vi "Curtin1_Acquire.vi"(8 "MainVI":refnum<vi>, 11 "Settings":T3={"Name of test"="ScratchPad", "Date"=timestamp(0 s since 1904-01-01), "Location"="Home", "Template"="ScratchPad", "Soundcard"="OCTA-CAPTURE", "resolution"=32, "Sampling rate"=48000, "Ch1 Gain "=25.0, "Ch2 Gain"=10.0, "Sample time (s)"=0.3, "Pre-trigger (s)"=0.001, "Hammer Threshold"=10.0, "Positions"=12, "Taps/Position"=5, "Set Names"="H,V", "Freq resolution"=1.0, "Hammer cutoff"=0.025, "Mic cutoff"=0.25, "Double bounce "=10.0, "Hammer Cal"=10.0, "dB Offset"=0.0, "Accel Cal"=10.0, "Vibrometer Cal"=0.0, "Mic Cal"=0.0, "Output"=2, "Voltage Cal"=0.01, "Vibrometer Port"="ASRL27::INSTR", "Range"=4, "High Pass"=2, "Bandwidth"=4, "X Range"=[], "Y Range"=[], "dB Spread"=0.0, "Trigger"=0, "Ch_1"=25, "Ch_2"=25, "flip?"=FALSE, "60Hz"=FALSE, "Time offset"=0.0, "Piezo Cal"=1.0, "Default Notes"=""} {"Ch_2" min=1 step=1; "Ch_1" min=1 max=100 step=1; "Trigger" items=["Hammer (force)", "Self-tap", "Spacebar"]; "Bandwidth" items=["1 kHz"=1, "5 kHz"=5, "10 kHz"=10, "25 kHz"=25, "50 kHz"=50, "100 kHz"=100]; "High Pass" items=["Off", "13 Hz", "104 Hz"]; "Range" items=["10 mm/s"=1, "20 mm/s"=2, "50 mm/s"=5, "100 mm/s"=10, "200 mm/s"=20, "500 mm/s"=50, "1 m/s"=100, "2 m/s"=200]; "Output" items=["Accelerometer", "Speed (from acceleration)", "Microphone", "Vibrometer", "Piezo"]; "Voltage Cal" format="%#_13g"; "Ch2 Gain" format="%#_13g"; "Ch1 Gain" format="%#_13g"; "Double bounce" min=0.0; "Mic cutoff" min=0.0 format="%#_4g"; "Hammer cutoff" min=0.0 format="%#_4g"; "Freq resolution" min=0.0; "Pre-trigger (s)" format="%#_13g"; "Date" format="%<%H:%M\n%d/%m/%y>T"; "resolution" items=["16 bit"=16, "24 bit"=24, "32 bit"=32]; "Sampling rate" items=["22050 samp/s"=22050, "44100 samp/s"=44100, "48000 samp/s"=48000]}) -> (1 "Name Change?":bool, 2 "Data?":bool, 3 "Average FRF":cluster{dbl, "df":dbl, dbl[]}[](graph))   [LabVIEW 2022 SP3]
uses:
  AmpCtrl.ctl
  PreferencesControl.ctl
  <extravilib>/ChannelInstances/Lossy Stream-a[.](wfm(dbl))/EndpointRead.vi
  Mic/Mic_Global.vi
  <extravilib>/ChannelInstances/Lossy Stream-a[.](wfm(dbl))/Instantiate.vi
  <extravilib>/ChannelInstances/Tag-a[.](wfm(dbl))/Instantiate.vi
  <extravilib>/ChannelInstances/Tag-a[.](wfm(dbl))/EndpointRead.vi
  <extravilib>/ChannelInstances/Lossy Stream-a[.](wfm(dbl))/)Channel.vi
  <resource>/ChannelSupport/_ChannelSupport/WaitIfNeeded.vi
  <extravilib>/ChannelInstances/Tag-a[.](wfm(dbl)).lvlib
  <extravilib>/ChannelInstances/Lossy Stream-a[.](wfm(dbl)).lvlib
panel:
  in  "Record Button":bool=TRUE
  in  "Tab Control":enum32{"graphs", "settings", "Notes"}(tab)
  in  "Move":bool
  in  "Motor Settings":bool
  in  "Tap":bool
  in  "Method":enum16{"Sqrt(H1H2)", "H1", "H2"}(ring)
  in  "History":bool=TRUE
  in  "Help":bool
  in  "Beam":bool
  in  "rescale Y Axes":bool
  in  "Open Sound":bool
  in  "View":u16(ring) items=["Raw", "Volts", "Units (Pa, N, etc)"]
  out "Hammer Spectrum":cluster{dbl, "df":dbl, "FFT {X}":dbl[]}[](graph)
  out "Hammer Data":cluster{dbl, "dt":dbl, "Y":dbl[]}[](graph)
  out "Microphone Data":cluster{dbl, "dt":dbl, "Y":dbl[]}[](graph)
  out "Volume":T1 {"Mic" scale=0.0..100.0; "Hammer" scale=0.0..100.0}
  in  "OpenVibrometer":bool
  in  "New":bool
  in  "Save SP":bool
  in  "Export":bool
  in  "Plot View":T2={"Alerts"=FALSE, "Log X Axis"=TRUE, "dB scale"=TRUE, "Averaging"=TRUE, "Fade"=0.0, "Centroids?"=FALSE}
  in  "Locked":bool
  in  "Notes":string
  in  "Done":bool
  out "Progress Bar":picture
  in  "zoom":bool
  in  "dB Spread":dbl=40.0
  in  "rescale Y":bool
  in  "stop":bool
  out "Alarms":string
  # "Hz"
  # "dB"
  # "dB"
  # "sec"
  # "sec"
  # "mV/Pa"
  # "mV/m/s2"
  # "mV/mm/s"
  # "V/N"
  # "sec"
  # "sec"
  # "mV/N"
  # "a.u."
  # "a.u."
  # "sec"
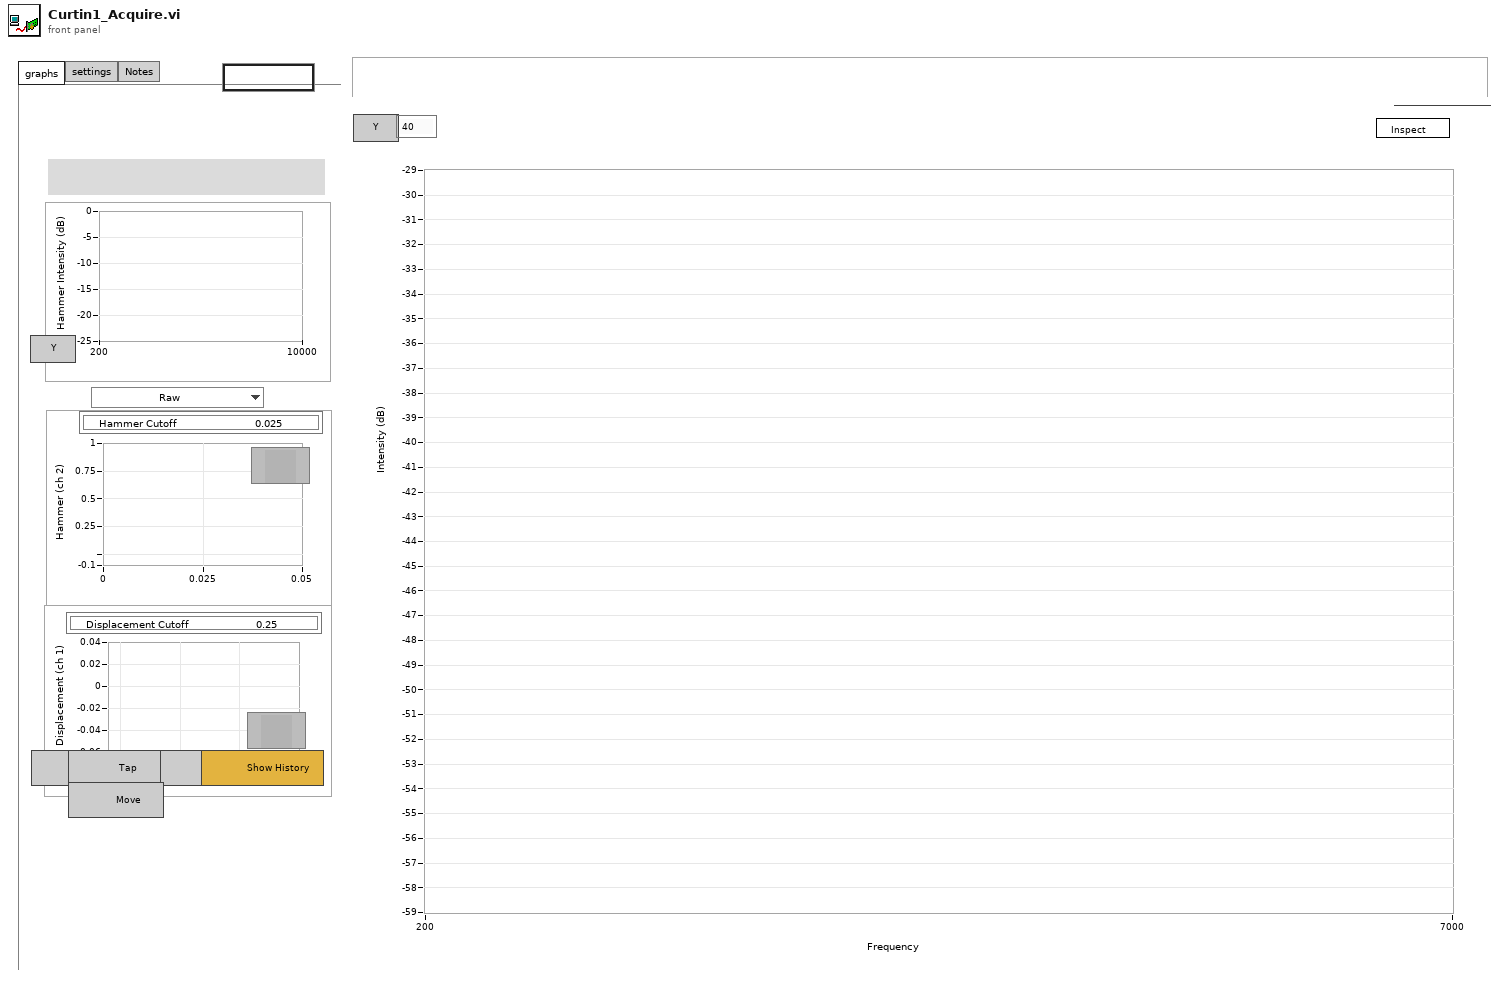
[diagram p1: front panel]
types:
  T1 = typedef "AmpCtrl.ctl" = cluster{"Hammer":u8, "Mic":u8, "Mic In":string}
  T2 = cluster{"Alerts":bool, "Log X Axis":bool, "dB scale":bool, "Averaging":bool, "Fade":dbl, "Centroids?":bool}
  T3 = typedef "PreferencesControl.ctl" = cluster{"Name of test":string, "Date":timestamp, "Location":string, "Template":string, "Soundcard":string, "resolution":u16, "Sampling rate":u16, "Ch1 Gain ":dbl, "Ch2 Gain":dbl, "Sample time (s)":dbl, "Pre-trigger (s)":dbl, "Hammer Threshold":dbl, "Positions":i16, "Taps/Position":i16, "Set Names":string, "Freq resolution":dbl, "Hammer cutoff":dbl, "Mic cutoff":dbl, "Double bounce ":dbl, "Hammer Cal":dbl, "dB Offset":dbl, "Accel Cal":dbl, "Vibrometer Cal":dbl, "Mic Cal":dbl, "Output":u16, "Voltage Cal":dbl, "Vibrometer Port":refnum<visa-resource-name>, "Range":u16, "High Pass":u16, "Bandwidth":u16, "X Range":cluster{"Minimum":dbl, "Maximum":dbl, "Increment":dbl, "Minor Increment":dbl, "Start":dbl}[], "Y Range":cluster{"Minimum":dbl, "Maximum":dbl, "Increment":dbl, "Minor Increment":dbl, "Start":dbl}[], "dB Spread":dbl, "Trigger":u16, "Ch_1":u8, "Ch_2":u8, "flip?":bool, "60Hz":bool, "Time offset":dbl, "Piezo Cal":dbl, "Default Notes":string}
  T4 = enum32{"Invalid", "Standard", "Closed", "Hidden", "Minimized", "Maximized"}
  T5 = enum16{"Initialize", "Free run", "One Shot - waiting", "One Shot - triggered", "Wait", "Close"}
  T6 = enum16{"Always On", "Always Off", "Off While Running"}
  T7 = enum8{"Enabled", "Disabled", "Disabled and Grayed Out"}
  T8 = typedef "Tag-a[.](wfm(dbl)).lvlib/))Channel.ctl" = refnum<queue>
  T9 = typedef "Lossy Stream-a[.](wfm(dbl)).lvlib/)Channel.ctl" = refnum<queue>
  T10 = typedef "LVBoundsTypeDef.ctl" = cluster{"Width":u32, "Height":u32}
  T11 = cluster{"Minimum":dbl, "Maximum":dbl, "Increment":dbl, "Minor Increment":dbl, "Start":dbl}
  T12 = typedef "eventvkey.ctl" = enum16{"ASCII", "Enter", "Return", "Shift", "Ctrl", "Alt", "Cmd", "Opt", "Caps", "NumLock", "Clear", "Break", "Up", "Down", "Left", "Right", "Insert", "Delete", "Home", "End", "PageUp", "PageDown", "Escape", "Help", "Pause", "ScrollLock", "F1", "F2", "F3", "F4", "F5", "F6", "F7", "F8", "F9", "F10", "F11", "F12", "F13", "F14", "F15", "F16", "F17", "F18", "F19", "F20", "F21", "F22", "F23", "F24", "Play", "VolumeUp", "VolumeDown", "Mute", "Two Byte Char"}
  T13 = typedef "LVMouseTypeDef.ctl" = cluster{"Mouse Position":cluster{"X":i32, "Y":i32}, "Mouse Modifiers":cluster{"Button Down":bool, "Shift Mod":bool, "Menu Mod":bool, "Option Mod":bool}}
  T14 = typedef "LVRangeTypeDef.ctl" = cluster{"Minimum":dbl, "Maximum":dbl, "Increment":dbl, "Minor Increment":dbl, "Start":dbl}
  T15 = cluster{"Minimum":dbl, "Maximum":dbl, "Increment":dbl, "Minor Increment":dbl, "Start":dbl}[]
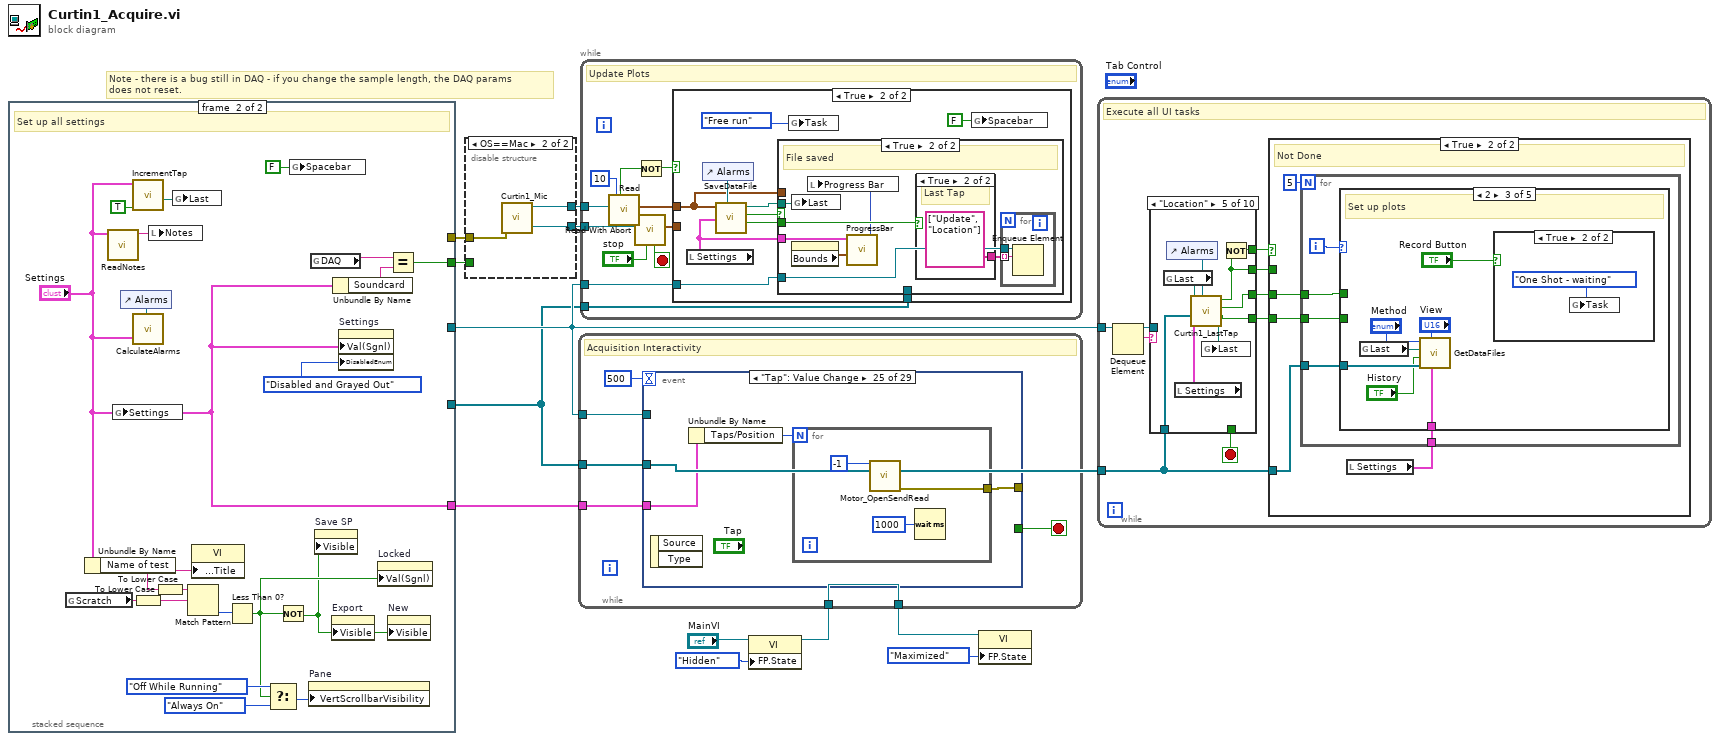
[diagram p0: block diagram]
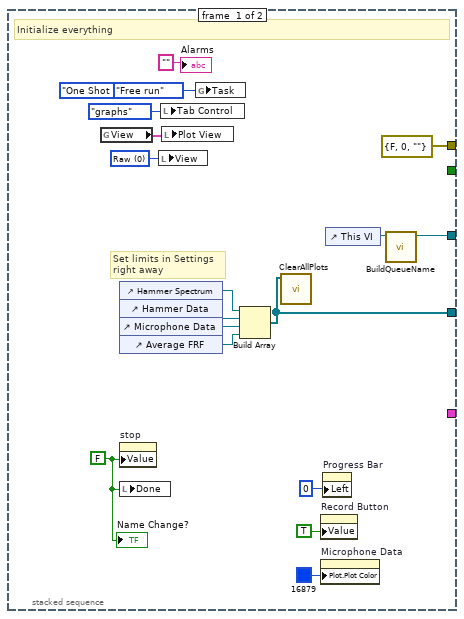
[diagram p2: hidden frame]
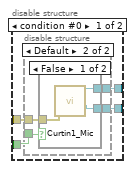
[diagram p3: hidden frame]
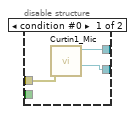
[diagram p4: hidden frame]
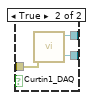
[diagram p5: hidden frame]
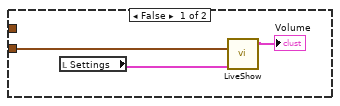
[diagram p6: hidden frame]
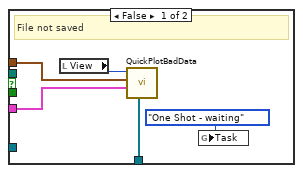
[diagram p7: hidden frame]
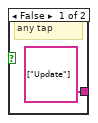
[diagram p8: hidden frame]
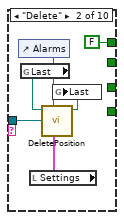
[diagram p10: hidden frame]
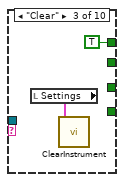
[diagram p11: hidden frame]
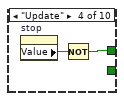
[diagram p12: hidden frame]
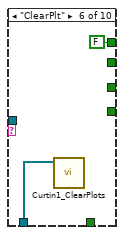
[diagram p13: hidden frame]
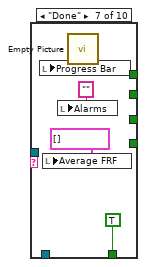
[diagram p14: hidden frame]
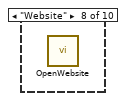
[diagram p15: hidden frame]
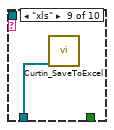
[diagram p16: hidden frame]
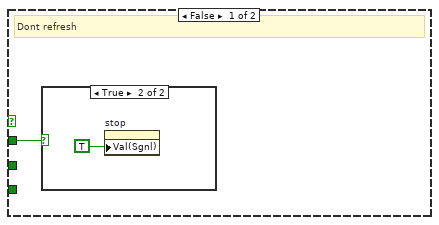
[diagram p18: hidden frame]
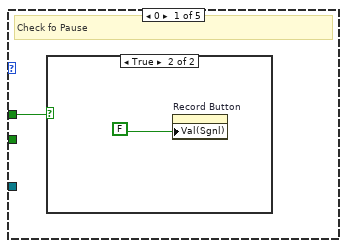
[diagram p20: hidden frame]
diagram:
  # "Note - there is a bug still in DAQ - if you change the sample length, the DAQ params \ndoes not reset."
  n1 = stacked-sequence {
    tunnel: [_ "Settings"] -> w5
    tunnel: [_ w39] -> w4
    tunnel: [w19 _] -> w3
    tunnel: [errorcluster {"status"=FALSE, "code"=0, "source"=""} ("error in (no error)") _] -> w2
    tunnel: [w13 _] -> w1
    frame #0 {
      w26 = u16 0 items=["Raw", "Volts", "Units (Pa, N, etc)"] ("View")
      w28 = FALSE ("stop")
      # "Set limits in Settings \nright away"
      # "Initialize everything"
      n2 = global read "Mic_Global.vi" "View"() -> (w29:T2)
      n3 = control-ref of="Hammer Spectrum"() -> (w14:refnum<vi>)
      n4 = control-ref of="Hammer Data"() -> (w15:refnum<vi>)
      n5 = control-ref of="Microphone Data"() -> (w16:refnum<vi>)
      n6 = control-ref of="Average FRF"() -> (w17:refnum<vi>)
      n7 = property on="stop" class="Bool (strict)"("Value"=w28) -> ()  [unwired: 2 in, 2 out]
      n8 = local write "Done"(w28) -> ()
      n9 = local write "View"(w26) -> ()
      n10 = local write "Tab Control"(enum32{"graphs", "settings"}."graphs" ("Tab Control")) -> ()
      n11 = local write "Plot View"(w29) -> ()
      n12 = global write "Mic_Global.vi" "Task"(T5."One Shot - waiting" ("Task")) -> ()
      n13 = global write "Mic_Global.vi" "Task"(T5."Free run" ("Task")) -> ()
      n14 = Build Array(w14, w15, w16, w17) -> (w13:refnum<vi>[])
      n15 = call "ClearAllPlots.vi"("Array"=w13) -> ()  [unwired: 11 in]
      n16 = property on="Record Button" class="Bool (strict)"("Value"=TRUE ("Good point?")) -> ()  [unwired: 2 in, 2 out]
      n17 = property on="Microphone Data" class="WFGraph (strict)"("Plot.Plot Color"=u32 16879) -> ()  [unwired: 2 in, 2 out]
      n18 = property on="Progress Bar" class="Pict"("Left"=i16 0 ("Origin:Left")) -> ()  [unwired: 2 in, 2 out]
      n19 = control-ref of="This VI"() -> (w20:refnum<vi>)
      n20 = call "BuildQueueName.vi"("VI in"=w20) -> ("Queue out"=w19:refnum<queue>)  [unwired: 9 in, 1 out]
      "Name Change?" <- w28
      "Alarms" <- "" ("Alarms")
    }
    frame #1 {
      # "Set up all settings"
      n21 = global read "Mic_Global.vi" "Scratch"() -> (w45:string)
      n22 = Unbundle By Name("Settings") -> ("Name of test"=w44:string)
      n23 = call "ReadNotes.vi"("Settings"="Settings") -> ("Notes"=w49:string)  [unwired: 9 in, 1 out]
      n24 = global write "Mic_Global.vi" "Settings"("Settings") -> ()
      n25 = control-ref of="Alarms"() -> (w46:refnum<vi>)
      n26 = call "IncrementTap.vi"("Reset?"=TRUE, "Settings"="Settings") -> ("Last Data Set"=w48:path)  [unwired: 4 in, 5 out]
      n27 = call "CalculateAlarms.vi"("Settings"="Settings", "Alarm"=w46) -> ()  [unwired: 8 in, 2 out]
      n28 = To Lower Case(string=w45) -> (all lower case string=w32:string)
      n29 = local write "Notes"(w49) -> ()
      n30 = To Lower Case(string=w44) -> (all lower case string=w33:string)
      n31 = global write "Mic_Global.vi" "Last"(w48) -> ()
      n32 = Match Pattern(string=w33, regular expression=w32) -> (offset past match=w43:i32)  [unwired: 1 in, 3 out]
      n33 = property class="VI"("Front Panel.Title"=w44) -> ()  [unwired: 2 in, 2 out]
      n34 = Less Than 0?(x=w43) -> (x < 0?=w35:bool)
      n35 = Select(t=T6."Off While Running" ("Vertical Scrollbar Visibility"), s=w35, f=T6."Always On" ("Vertical Scrollbar Visibility")) -> (s? t:f=w42:T6)
      n36 = Not(x=w35) -> (.not. x?=w34:bool)
      n37 = global write "Mic_Global.vi" "Spacebar"(FALSE ("Spacebar")) -> ()
      n38 = property on="Pane" class="Pane"("VertScrollbarVisibility"=w42) -> ()  [unwired: 2 in, 2 out]
      n39 = global read "Mic_Global.vi" "DAQ"() -> (w41:string)
      n40 = property on="Save SP" class="Bool"("Visible"=w34) -> ()  [unwired: 2 in, 2 out]
      n41 = property on="Export" class="Bool"("Visible"=w34) -> ()  [unwired: 2 in, 2 out]
      n42 = Unbundle By Name("Settings") -> ("Soundcard"=w40:string)
      n43 = property on="Settings" class="Clust (strict)"("Val(Sgnl)"="Settings", "DisabledEnum"=T7."Disabled and Grayed Out" ("Disabled")) -> ()  [unwired: 2 in, 2 out]
      n44 = property on="Locked" class="Bool (strict)"("Val(Sgnl)"=w35) -> ()  [unwired: 2 in, 2 out]
      n45 = Equal?(x=w41, y=w40) -> (x = y?=w39:bool)
      n46 = property on="New" class="Bool"("Visible"=w34) -> ()  [unwired: 2 in, 2 out]
    }
  }
  n47 = disable-structure shown="OS==Mac" {
    disable-tunnel: w2 -> [w54 w70]
    disable-tunnel: [w53 w68] -> w12
    disable-tunnel: [w52 w69] -> w11
    disable-tunnel: w4 -> [w51 _]
    frame condition #0 {
      n48 = disable-structure shown="Default" {
        disable-tunnel: w54 -> [w55 w59]
        disable-tunnel: [w57 w61] -> w53
        disable-tunnel: [w56 w60] -> w52
        disable-tunnel: w51 -> [_ w58]
        frame condition #0 {
          n49 = call "Curtin1_Mic.vi"("error in (no error)"=w55) -> ("latest data"=w57:T8, "Tap"=w56:T9)  [unwired: 9 in]
        }
        frame condition #1 (active) {
          n50 = case shown="False" w58 {
            tunnel: [w63 w67] -> w61
            tunnel: [w62 w66] -> w60
            tunnel: w59 -> [w64 w65]
            frame False {
              n51 = call "Curtin1_Mic.vi"("error in (no error)"=w64) -> ("latest data"=w63:T8, "Tap"=w62:T9)  [unwired: 9 in]
            }
            frame True {
              n52 = call "Curtin1_DAQ.vi"("error in (no error)"=w65) -> ("Buffer"=w67:T8, "Tap"=w66:T9)  [unwired: 9 in]
            }
          }
        }
      }
    }
    frame condition #1 (active) {
      n53 = call "Curtin1_Mic.vi"("error in (no error)"=w70) -> ("latest data"=w68:T8, "Tap"=w69:T9)  [unwired: 9 in]
    }
  }
  n54 = while {
    tunnel: w11 -> [w81]
    tunnel: w12 -> [w78]
    tunnel: w3 -> [w72]
    tunnel: w1 -> [w71]
    stop <- w77 stop-if-true
    # "Update Plots"
    n55 = call <extravilib>:"Read.vi"("channel"=w81, "timeout in ms (-1)"=10) -> ("element"=w80:waveform(dbl)[], "timed out?"=w74:bool)  [unwired: 4 in, 4 out]
    n56 = call <extravilib>:"Read With Abort.vi"("abort"="stop", "channel"=w78) -> ("element"=w76:waveform(dbl)[], "aborted?"=w77:bool)  [unwired: 7 in, 1 out]
    n57 = Not(x=w74) -> (.not. x?=w73:bool)
    n58 = case shown="True" w73 {
      tunnel: w80 -> [_ w87]
      tunnel: w76 -> [w83 _]
      tunnel: w72 -> [_ w92]
      tunnel: w71 -> [_ w86]
      frame False {
        n59 = local read "Settings"() -> (w82:T3)
        n60 = call "LiveShow.vi"("Settings"=w82, "Buffer"=w83) -> ("Volume"=→"Volume":T1)  [unwired: 9 in]
      }
      frame True {
        n61 = local read "Settings"() -> (w88:T3)
        n62 = control-ref of="Alarms"() -> (w91:refnum<vi>)
        n63 = call "SaveDataFile.vi"("Settings"=w88, "Alarms"=w91, "Data"=w87) -> ("last tap?"=w93:bool, "New File?"=w94:bool, "new path"=w90:path)  [unwired: 4 in, 2 out]
        n64 = case shown="True" w94 {
          tunnel: w93 -> [_ w106]
          tunnel: w92 -> [_ w100]
          tunnel: w90 -> [_ w105]
          tunnel: w88 -> [w95 w103]
          tunnel: w87 -> [w96 _]
          tunnel: w86 -> [w97 _]
          frame False {
            # "File not saved"
            n65 = local read "View"() -> (w98:u16)
            n66 = call "QuickPlotBadData.vi"("Array"=w97, "Settings"=w95, "Data"=w96, "View"=w98) -> ()  [unwired: 8 in]
            n67 = global write "Mic_Global.vi" "Task"(T5."One Shot - waiting" ("Task")) -> ()
          }
          frame True {
            # "File saved"
            n68 = global write "Mic_Global.vi" "Last"(w105) -> ()
            n69 = property on="Progress Bar" class="Pict"() -> ("Bounds"=w101:T10)  [unwired: 2 in, 2 out]
            n70 = call "ProgressBar.vi"("Bounds"=w101, "Settings"=w103) -> ("Progress Bar"=w102:picture)  [unwired: 7 in, 2 out]
            n71 = local write "Progress Bar"(w102) -> ()
            n72 = case shown="True" w106 {
              tunnel: [string[] ["Update"] string[] ["Update", "Location"]] -> w104
              frame False {
                # "any tap"
              }
              frame True {
                # "Last Tap"
              }
            }
            n73 = for {
              tunnel: w104 -> [w108] mode=indexing
              tunnel: w100 -> [w107]
              n74 = Enqueue Element(queue=w107, element=w108) -> ()  [unwired: 2 in, 3 out]
            }
          }
        }
        n75 = global write "Mic_Global.vi" "Task"(T5."Free run" ("Task")) -> ()
        n76 = global write "Mic_Global.vi" "Spacebar"(FALSE ("Spacebar")) -> ()
      }
    }
  }
  n77 = property class="VI"(reference="MainVI", "FP.State"=T4."Hidden" ("Front Panel Window:State")) -> (reference out=w6:refnum<vi>)  [unwired: 1 in, 1 out]
  n78 = while {
    tunnel: w1 -> [w116]
    tunnel: w3 -> [w113]
    tunnel: [w112] -> w7
    tunnel: w6 -> [w112]
    tunnel: w5 -> [w111]
    stop <- w114 stop-if-true
    # "Acquisition Interactivity"
    n79 = event shown="[24] \"Tap\": Value Change" {
      selector: _ -> [_ _ _ _ _ _ _ _ _ _ _ _ _ _ _ _ _ _ _ _ _ _ _ _ _ _ _ _ _]
      dyn-events: _ -> [_ _ _ _ _ _ _ _ _ _ _ _ _ _ _ _ _ _ _ _ _ _ _ _ _ _ _ _ _]
      timeout: 500 -> [_ _ _ _ _ _ _ _ _ _ _ _ _ _ _ _ _ _ _ _ _ _ _ _ _ _ _ _ _]
      tunnel: [_ _ _ _ _ _ _ _ _ _ _ _ _ _ _ _ _ _ _ w246 _ _ _ _ _ _ _ _ w277] -> w114
      tunnel: w116 -> [w120 w132 _ _ _ w151 _ _ _ _ _ _ _ w192 _ _ _ _ _ _ _ _ _ _ _ _ _ _ _]
      tunnel: w113 -> [_ _ _ _ _ w155 _ w161 w166 w176 w183 w186 _ w191 _ _ _ _ _ w245 _ _ _ _ _ _ _ _ w276]
      tunnel: [_ _ _ _ _ _ _ _ _ _ _ _ _ _ _ _ _ _ w231 _ _ _ _ _ w266 w272 _ _ _] -> _
      tunnel: w111 -> [_ _ _ _ _ _ _ _ _ _ _ _ _ _ _ _ w221 _ _ w241 _ _ w262 _ w265 _ _ _ _]
      event "Hammer Data", "Microphone Data", "Average FRF", "Hammer Spectrum": Mouse Up {
        n80 = event-data() -> ("PlatMods.Shift"=w121:bool, "CtlRef"=w119:refnum<vi>)  [unwired: 1 in]
        n81 = local read "History"() -> (w123:bool)
        n82 = Search 1D Array(1D array=w120, element=w119) -> (index of element=w118:i32)  [unwired: 1 in]
        n83 = case shown="1, 2" w118 {
          tunnel: [9 0] -> w117
          frame 1, 2 {
          }
          frame Default {
          }
        }
        n84 = call "BuildZoomNames.vi"("History"=w123, "WaveformGraph in"=w119) -> ("Names"=w122:string[])  [unwired: 9 in]
        n85 = case shown="True" w121 {
          tunnel: w119 -> [_ w129]
          tunnel: w122 -> [_ w127]
          tunnel: w117 -> [_ w126]
          frame False {
          }
          frame True {
            n86 = local read "dB Spread"() -> (w128:dbl)
            n87 = call "GraphZoom.vi"("Plot"=w126, "Names"=w127, "dB Range"=w128, "Graph"=w129) -> ()  [unwired: 8 in]
          }
        }
      }
      event "zoom": Value Change {
        n88 = event-data() -> ()  [unwired: 1 in, 1 out]
        n89 = Index Array(array=w132, index=3) -> (element=w130:refnum<vi>)
        n90 = local read "History"() -> (w135:bool)
        n91 = call "BuildZoomNames.vi"("History"=w135, "WaveformGraph in"=w130) -> ("Names"=w134:string[])  [unwired: 9 in]
        n92 = local read "dB Spread"() -> (w133:dbl)
        n93 = call "GraphZoom.vi"("Names"=w134, "dB Range"=w133, "Graph"=w130) -> ()  [unwired: 9 in]
      }
      event "Microphone Data": Cursor Move {
        n94 = event-data() -> ("CursLoc.X"=w136:dbl)  [unwired: 1 in]
        n95 = property on="Mic cutoff" class="DigNum (strict)"("Val(Sgnl)"=w136) -> ()  [unwired: 2 in, 2 out]
      }
      event "Hammer Data": Cursor Move {
        n96 = event-data() -> ("CursIdx"=w138:i32, "CursLoc.X"=w139:dbl, "CursLoc.Y"=w137:dbl)  [unwired: 1 in]
        n97 = case shown="0" w138 {
          tunnel: w139 -> [w140 _]
          tunnel: w137 -> [_ w141]
          frame 0 {
            n98 = property on="Hammer cutoff" class="DigNum (strict)"("Val(Sgnl)"=w140) -> ()  [unwired: 2 in, 2 out]
          }
          frame Default {
            n99 = property on="Hammer Threshold" class="DigNum (strict)"("Val(Sgnl)"=w141) -> ()  [unwired: 2 in, 2 out]
          }
        }
      }
      event "Notes": Value Change {
        n100 = event-data() -> ()  [unwired: 1 in, 1 out]
        n101 = local read "Settings"() -> (w143:T3)
        n102 = call "Curtin1_SaveNotesFile.vi"("Notes"="Notes", "Settings in"=w143) -> ()  [unwired: 10 in]
      }
      event Value Change {
        n103 = event-data() -> ("NewVal"=w149:T3, "OldVal"=w148:T3)  [unwired: 1 in]
        n104 = Enqueue Element(queue=w155, element="Update") -> ()  [unwired: 2 in, 3 out]
        n105 = call "VibrometerSettings.vi"("OldVal"=w148, "NewVal"=w149) -> ("Settings"=w144:T3)  [unwired: 6 in, 3 out]
        n106 = global write "Mic_Global.vi" "Settings"(w144) -> ()
        n107 = call "Curtin1_SaveLastSettingsFile.vi"("Settings in"=w144) -> ()  [unwired: 11 in]
        n108 = call "Curtin1_updatePlots.vi"("plots"=w151, "Settings"=w144) -> ()  [unwired: 10 in]
        n109 = Unbundle By Name(w144) -> ("dB Spread"=w150:dbl, "Output"=w146:u16)
        n110 = call "Read_Write_Test_Parameters.vi"("Task"=enum16{"Save", "Read", "Clear"}."Save", "Settings"=w144) -> ("Settings"=w152:T3)  [unwired: 8 in, 1 out]
        n111 = local write "dB Spread"(w150) -> ()
        n112 = call "IncrementTap.vi"("Settings"=w152) -> ("Last Data Set"=w153:path)  [unwired: 5 in, 5 out]
        n113 = Equal?(x=u16 3 ("Output"), y=w146) -> (x = y?=w145:bool)
        n114 = global write "Mic_Global.vi" "Last"(w153) -> ()
        n115 = property on="Beam" class="Bool (strict)"("Visible"=w145) -> ()  [unwired: 2 in, 2 out]
      }
      event "dB Spread": Value Change {
        n116 = event-data() -> ("NewVal"=w158:dbl)  [unwired: 1 in]
        n117 = local read "Settings"() -> (w159:T3)
        n118 = Bundle By Name(cluster=w159, "dB Spread"=w158) -> (w157:T3)
        n119 = local write "Settings"(w157) -> ()
        n120 = global write "Mic_Global.vi" "Settings"(w157) -> ()
      }
      event Key Up {
        n121 = event-data() -> ("ScanCode"=w163:i16, "PlatMods.Shift"=w162:bool)  [unwired: 1 in]
        n122 = call "Check KeyUp.vi"("Shift"=w162, "ScanCode"=w163) -> ("Task"=w160:string)  [unwired: 9 in]
        n123 = case shown="\"\"" w160 {
          selector: w160 -> [_ w164]
          tunnel: w161 -> [_ w165]
          frame "" {
          }
          frame Default {
            n124 = Enqueue Element(queue=w165, element=w164) -> ()  [unwired: 2 in, 3 out]
          }
        }
      }
      event Key Down {
        n125 = event-data() -> ("VKey"=w167:T12)  [unwired: 1 in, 3 out]
        n126 = case shown="\"Left\", \"Right\"" w167 {
          selector: w167 -> [_ w171]
          tunnel: w166 -> [_ w168]
          frame "ASCII", Default {
          }
          frame "Left", "Right" {
            n127 = Format Into String(w171) -> (resulting string=w170:string)  [unwired: 3 in, 1 out]
            n128 = Enqueue Element(queue=w168, element="Update") -> ()  [unwired: 2 in, 3 out]
            n129 = call "FadeLeftRight.vi"("Key"=w170) -> ()  [unwired: 11 in]
          }
        }
      }
      event "Progress Bar": Mouse Up {
        # "need to end free run\nif in Done condition"
        n130 = event-data() -> ()  [unwired: 1 in, 1 out]
        n131 = property on="Progress Bar" class="Pict"() -> ("Mouse"=w177:T13, "Bounds"=w175:T10)  [unwired: 2 in, 2 out]
        n132 = local read "Settings"() -> (w174:T3)
        n133 = global write "Mic_Global.vi" "Task"(T5."Free run" ("Task")) -> ()
        n134 = call "DetermineSetChosen.vi"("Settings"=w174, "Bounds"=w175, "Mouse"=w177) -> ("Queue Task"=w172:string)  [unwired: 7 in, 1 out]
        n135 = case shown="Default" w172 {
          selector: w172 -> [_ w178]
          tunnel: w176 -> [_ w181]
          tunnel: w174 -> [_ w180]
          frame "" {
          }
          frame Default {
            n136 = Enqueue Element(queue=w181, element=w178) -> ()  [unwired: 2 in, 3 out]
            n137 = control-ref of="Alarms"() -> (w179:refnum<vi>)
            n138 = call "CalculateAlarms.vi"("Settings"=w180, "Alarm"=w179) -> ()  [unwired: 8 in, 2 out]
          }
        }
      }
      event "Plot View": Value Change {
        n139 = event-data() -> ()  [unwired: 1 in, 4 out]
        n140 = Enqueue Element(queue=w183, element="Update") -> ()  [unwired: 2 in, 3 out]
        n141 = global write "Mic_Global.vi" "View"("Plot View") -> ()
      }
      event "View", "History", "Method": Value Change {
        n142 = event-data() -> ()  [unwired: 1 in, 4 out]
        n143 = Enqueue Element(queue=w186, element="Update") -> ()  [unwired: 2 in, 3 out]
      }
      event "Record Button": Value Change {
        n144 = event-data() -> ("NewVal"=w187:bool)  [unwired: 1 in]
        n145 = Select(t=T5."One Shot - waiting" ("Task"), s=w187, f=T5."Free run" ("Task")) -> (s? t:f=w189:T5)
        n146 = global write "Mic_Global.vi" "Task"(w189) -> ()
      }
      event "Average FRF", "Hammer Spectrum", "Microphone Data", "Hammer Data": Scale Range Change; "rescale Y": Value Change {
        n147 = event-data() -> ()  [unwired: 1 in, 1 out]
        n148 = stacked-sequence {
          tunnel: w192 -> [w194 w205 _]
          tunnel: w191 -> [_ _ w206]
          frame #0 {
            n149 = case shown="False" "rescale Y" {
              tunnel: w194 -> [_ w200]
              tunnel: "dB Spread" -> [_ w197]
              frame False {
              }
              frame True {
                n150 = Index Array(array=w200, index=3) -> (element=w198:refnum<vi>)
                n151 = call "AutoscaleYaxis.vi"("Has Coherence in plot?"=TRUE, "dB Range"=w197, "WaveformGraph in"=w198) -> ()  [unwired: 9 in]
              }
            }
          }
          frame #1 {
            n152 = call "GetPlotRanges.vi"("plots"=w205) -> ("Yscales"=w202:T14[], "Xscales"=w203:T14[])  [unwired: 9 in]
            n153 = local read "Settings"() -> (w204:T3)
            n154 = Bundle By Name(cluster=w204, "X Range"=w203, "Y Range"=w202) -> (w201:T3)
            n155 = property on="Settings" class="Clust (strict)"("Val(Sgnl)"=w201) -> ()  [unwired: 2 in, 2 out]
          }
          frame #2 {
            # "done in settings update"
            n156 = disable-structure shown="Disabled" {
              disable-tunnel: w206 -> [w207 _]
              frame Disabled {
                n157 = Enqueue Element(queue=w207, element="Update") -> ()  [unwired: 2 in, 3 out]
              }
              frame Enabled {
              }
            }
          }
        }
      }
      event "Locked": Value Change {
        n158 = event-data() -> ()  [unwired: 1 in, 1 out]
        n159 = property on="Export" class="Bool"() -> ("Visible"=w212:bool)  [unwired: 2 in, 2 out]
        n160 = Not(x=w212) -> (.not. x?=w211:bool)
        n161 = Not(x="Locked") -> (.not. x?=w209:bool)
        n162 = Select(t=T7."Disabled and Grayed Out" ("Disabled"), s="Locked", f=T7."Enabled" ("Disabled")) -> (s? t:f=w215:T7)
        n163 = And(x=w209, y=w211) -> (x .and. y?=w210:bool)
        n164 = property on="Settings" class="Clust (strict)"("DisabledEnum"=w215) -> ()  [unwired: 2 in, 2 out]
        n165 = property on="Save SP" class="Bool"("Visible"=w209) -> ()  [unwired: 2 in, 2 out]
        n166 = case shown="True" w210 {
          tunnel: "Warning: You should not edit these parameters in the middle of a run.  Instead, play around in ScratchPad and then Export your new settings as a template." -> [_ w218]
          frame False {
          }
          frame True {
            n167 = One Button Dialog(message=w218) -> ()  [unwired: 1 in, 1 out]
          }
        }
      }
      event "Export": Value Change {
        n168 = event-data() -> ()  [unwired: 1 in, 3 out]
        n169 = local read "Settings"() -> (w219:T3)
        n170 = call "Curtin_SaveTemplate.vi"("Settings in"=w219) -> ()  [unwired: 8 in, 3 out]
      }
      event "Save SP": Value Change {
        n171 = event-data() -> ()  [unwired: 1 in, 1 out]
        n172 = local read "Settings"() -> (w222:T3)
        n173 = call "CheckForTemplateEdits.vi"("Original Settings"=w221, "Force?"=TRUE, "Current Settings"=w222) -> ()  [unwired: 8 in, 1 out]
      }
      event "New": Value Change {
        n174 = event-data() -> ()  [unwired: 1 in, 3 out]
        n175 = local read "Settings"() -> (w227:T3)
        n176 = local write "Name Change?"(TRUE ("Name Change?")) -> ()
        n177 = property on="Record Button" class="Bool (strict)"("Value"=FALSE ("Good point?")) -> ()  [unwired: 2 in, 2 out]
        n178 = call "RenameScratchtoTest.vi"("Settings"=w227) -> ("Ok?"=w228:bool, "Name of test"=w225:string, "Settings Out"=w224:T3)  [unwired: 8 in]
        n179 = case shown="True" w228 {
          tunnel: w225 -> [_ w230]
          tunnel: w224 -> [_ w229]
          frame False {
          }
          frame True {
            n180 = local write "Settings"(w229) -> ()
            n181 = global write "Mic_Global.vi" "Settings"(w229) -> ()
            n182 = property class="VI"("Front Panel.Title"=w230) -> ()  [unwired: 2 in, 2 out]
          }
        }
      }
      event "Open Sound": Value Change {
        # "F1 will open this"
        n183 = event-data() -> ()  [unwired: 1 in, 3 out]
        n184 = Open VI Reference(vi path="Curtin1_Mic.vi") -> (vi reference=w234:refnum<vi>, error out=w232:errorcluster)  [unwired: 5 in]
        n185 = invoke class="VI" method="FP.Open"(reference=w234, error in=w232, "Activate"=TRUE ("Activate?")) -> (error out=w231:errorcluster)  [unwired: 2 in, 4 out]
      }
      event "stop": Value Change {
        w243 = cluster{dbl, "df":dbl, dbl[]}[] [] ("Average FRF")
        # "Do not ask if you only changed axis ranges"
        n186 = event-data() -> ("NewVal"=w246:bool)  [unwired: 1 in]
        n187 = call "Read_Write_Test_Parameters.vi"("Task"=enum16{"Save", "Read", "Clear"}."Read", "Settings"=w241) -> ("Settings"=w240:T3)  [unwired: 8 in, 1 out]
        n188 = local read "Settings"() -> (w238:T3)
        n189 = Enqueue Element(queue=w245, element="Done") -> ()  [unwired: 2 in, 3 out]
        n190 = call "CheckForTemplateEdits.vi"("Original Settings"=w240, "Force?"=FALSE, "Current Settings"=w238) -> ("Current Settings out"=w236:T3)  [unwired: 8 in]
        n191 = global write "Mic_Global.vi" "Settings"(w238) -> ()
        n192 = call "CheckScratchAndExit.vi"("Settings"=w236) -> ("Ask?"=→"Data?":bool)  [unwired: 10 in]
        "Microphone Data" <- w243
        "Hammer Data" <- w243
        "Hammer Spectrum" <- w243
        "Average FRF" <- w243
      }
      event "rescale Y Axes": Value Change {
        n193 = event-data() -> ()  [unwired: 1 in, 1 out]
        n194 = local read "Settings"() -> (w248:T3)
        n195 = Unbundle By Name(w248) -> ("Y Range"=w247:T15, "Trigger"=w249:u16)
        n196 = case shown="0, Default" w249 {
          tunnel: w248 -> [w256 _]
          tunnel: w247 -> [w251 _]
          frame 0, Default {
            n197 = Replace Array Subset(array=w251, new element #1=T11 {"Minimum"=-0.1, "Maximum"=1.0, "Increment"=0.2, "Minor Increment"=0.05, "Start"=0.0} ("XScale.Range"), index #1=1 ("index"), new element #2=T11 {"Minimum"=-1.0, "Maximum"=1.0, "Increment"=0.5, "Minor Increment"=0.1, "Start"=-1.0} ("XScale.Range")) -> (w250:T15)  [unwired: 1 in]
            n198 = Bundle By Name(cluster=w256, "Y Range"=w250) -> (w255:T3)
            n199 = property on="Settings" class="Clust (strict)"("Val(Sgnl)"=w255) -> ()  [unwired: 2 in, 2 out]
          }
          frame 1 {
            w257 = u8 1 ("Y Scale.Scale Fit")
            n200 = property on="Hammer Data" class="WFGraph (strict)"("YScale.ScaleFit"=w257) -> ()  [unwired: 2 in, 2 out]
            n201 = property on="Microphone Data" class="WFGraph (strict)"("YScale.ScaleFit"=w257) -> ()  [unwired: 2 in, 2 out]
          }
        }
      }
      event "Beam": Value Change {
        n202 = event-data() -> ()  [unwired: 1 in, 2 out]
        n203 = local read "Settings"() -> (w260:T3)
        n204 = Unbundle By Name(w260) -> ("Vibrometer Port"=w259:refnum<visa-resource-name>)
        n205 = call "Toggle Laser.vi"("Beam"="Beam", "RS232"=w259) -> ()  [unwired: 8 in, 2 out]
      }
      event "OpenVibrometer": Value Change {
        n206 = event-data() -> ()  [unwired: 1 in, 2 out]
        n207 = call "PolyTec_Control_Panel.vi"("Settings in"=w262) -> ("Settings Out"=w261:T3)  [unwired: 8 in, 2 out]
        n208 = property on="Settings" class="Clust (strict)"("Val(Sgnl)"=w261) -> ()  [unwired: 2 in, 2 out]
      }
      event "Motor Settings": Value Change {
        n209 = event-data() -> ()  [unwired: 1 in, 2 out]
        n210 = case shown="True" "Motor Settings" {
          frame False {
          }
          frame True {
            n211 = call "MotorControl.vi"() -> ()  [unwired: 12 in]
          }
        }
      }
      event "Tap": Value Change {
        n212 = event-data() -> ()  [unwired: 1 in, 2 out]
        n213 = Unbundle By Name(w265) -> ("Taps/Position"=w264:i16)
        n214 = for {
          N: w264 -> [_]
          tunnel: [w269] -> w266
          n215 = call "Motor_OpenSendRead.vi"("Angle to move"=-1) -> ("error out"=w269:errorcluster)  [unwired: 8 in, 2 out]
          n216 = Wait (ms)(milliseconds to wait=u32 1000) -> ()  [unwired: 1 out]
        }
      }
      event "Move": Value Change {
        n217 = event-data() -> ()  [unwired: 1 in, 2 out]
        n218 = local read "Settings"() -> (w271:T3)
        n219 = call "Automation Control.vi"("Settings"=w271) -> ("desired position"=w270:dbl)  [unwired: 10 in]
        n220 = call "Motor_OpenSendRead.vi"("Angle to move"=w270) -> ("error out"=w272:errorcluster)  [unwired: 8 in, 2 out]
      }
      event "Help": Value Change {
        n221 = event-data() -> ()  [unwired: 1 in, 2 out]
        n222 = One Button Dialog(message="Hints:\n1. Cutoffs: Move the green lines to zero out noise data (replace acquired data with zero for all future times)\n2. Hammer trigger (purple line) lets you choose how hard the hammer has to hit to trigger a dataset\n3. click on Notes (at top) to add thoughts ") -> ()  [unwired: 1 in, 1 out]
      }
      event Panel Close? {
        n223 = event-data() -> ()  [unwired: 1 in, 1 out]
        n224 = property on="stop" class="Bool (strict)"("Val(Sgnl)"=TRUE ("Value (Signaling)")) -> ()  [unwired: 2 in, 2 out]
        n225 = event-data("Discard?"=TRUE) -> ()  [unwired: 1 in, 1 out]
      }
      event Timeout {
        n226 = event-data() -> ()  [unwired: 1 in, 1 out]
        n227 = case shown="True" "Done" {
          tunnel: [_ w281] -> w277
          tunnel: w276 -> [_ w280]
          frame False {
          }
          frame True {
            w281 = TRUE ("Value (Signaling)")
            n228 = Enqueue Element(queue=w280, element="Done") -> ()  [unwired: 2 in, 3 out]
            n229 = property on="stop" class="Bool (strict)"("Value"=w281) -> ()  [unwired: 2 in, 2 out]
          }
        }
      }
    }
  }
  n230 = property class="VI"(reference=w7, "FP.State"=T4."Maximized" ("Front Panel Window:State")) -> ()  [unwired: 1 in, 2 out]
  n231 = while {
    tunnel: w1 -> [w287]
    tunnel: w3 -> [w288]
    stop <- w289 stop-if-true
    # "Execute all UI tasks"
    n232 = Dequeue Element(queue=w288) -> (queue out=w283:refnum<queue>, element=w286:string)  [unwired: 2 in, 2 out]
    n233 = case shown="\"Location\"" w286 {
      tunnel: [_ FALSE TRUE w299 w305 FALSE _ _ _ _] -> w290
      tunnel: [_ _ _ _ _ _ TRUE _ _ _] -> w289
      tunnel: w287 -> [_ _ _ _ w309 w310 _ _ w316 _]
      tunnel: [_ _ _ _ w304 _ _ _ _ _] -> w285
      tunnel: [_ _ _ _ w302 _ _ _ _ _] -> w284
      tunnel: w283 -> [_ w293 _ _ _ _ _ _ _ _]
      tunnel: [_ _ _ _ w301 _ _ _ _ _] -> w282
      frame Default {
      }
      frame "Delete" {
        n234 = control-ref of="Alarms"() -> (w292:refnum<vi>)
        n235 = global read "Mic_Global.vi" "Last"() -> (w295:path)
        n236 = local read "Settings"() -> (w291:T3)
        n237 = call "DeletePosition.vi"("Settings"=w291, "Alarms"=w292, "queue"=w293, "last"=w295) -> ("Last Data Set"=w294:path)  [unwired: 6 in, 1 out]
        n238 = global write "Mic_Global.vi" "Last"(w294) -> ()
      }
      frame "Clear" {
        n239 = local read "Settings"() -> (w297:T3)
        n240 = call "ClearInstrument.vi"("Settings"=w297) -> ()  [unwired: 11 in]
      }
      frame "Update" {
        n241 = property on="stop" class="Bool (strict)"() -> ("Value"=w300:bool)  [unwired: 2 in, 2 out]
        n242 = Not(x=w300) -> (.not. x?=w299:bool)
      }
      frame "Location" {
        n243 = global read "Mic_Global.vi" "Last"() -> (w308:path)
        n244 = control-ref of="Alarms"() -> (w303:refnum<vi>)
        n245 = local read "Settings"() -> (w307:T3)
        n246 = call "Curtin1_LastTap.vi"("Alarms"=w303, "Plots"=w309, "Settings"=w307, "Data"=w308) -> ("Data Out"=w306:path, "New Set"=w304:bool, "Pause?"=w302:bool, "Done?"=w301:bool)  [unwired: 4 in]
        n247 = global write "Mic_Global.vi" "Last"(w306) -> ()
        n248 = Not(x=w301) -> (.not. x?=w305:bool)
      }
      frame "ClearPlt" {
        n249 = call "Curtin1_ClearPlots.vi"("Array"=w310) -> ()  [unwired: 11 in]
      }
      frame "Done" {
        n250 = local write "Average FRF"(cluster{dbl, "df":dbl, dbl[]}[] [] ("Average FRF")) -> ()
        n251 = local write "Alarms"("") -> ()
        n252 = call "Empty Picture"() -> ("empty picture"=w314:picture)
        n253 = local write "Progress Bar"(w314) -> ()
      }
      frame "Website" {
        n254 = call "OpenWebsite.vi"() -> ()  [unwired: 12 in]
      }
      frame "xls" {
        n255 = call "Curtin_SaveToExcel.vi"("plots"=w316) -> ()  [unwired: 11 in]
      }
      frame "Close" {
      }
    }
    n256 = case shown="True" w290 {
      tunnel: w287 -> [_ w322]
      tunnel: w285 -> [_ w321]
      tunnel: w284 -> [_ w320]
      tunnel: w282 -> [w317 _]
      frame False {
        # "Dont refresh"
        n257 = case shown="True" w317 {
          frame False {
          }
          frame True {
            n258 = property on="stop" class="Bool (strict)"("Val(Sgnl)"=TRUE ("Value (Signaling)")) -> ()  [unwired: 2 in, 2 out]
          }
        }
      }
      frame True {
        # "Not Done"
        n259 = local read "Settings"() -> (w319:T3)
        n260 = for {
          N: 5 ("timeout in ms (-1)") -> [_]
          tunnel: w322 -> [w327]
          tunnel: w321 -> [w326]
          tunnel: w320 -> [w325]
          tunnel: w319 -> [w324]
          i -> [w328]
          n261 = case shown="2" w328 {
            tunnel: w327 -> [_ _ w345 _ _]
            tunnel: w324 -> [_ w334 w343 w347 _]
            tunnel: w326 -> [_ _ _ _ _]
            tunnel: w325 -> [w329 _ _ _ _]
            frame 0 {
              # "Check fo Pause"
              n262 = case shown="True" w329 {
                frame False {
                }
                frame True {
                  n263 = property on="Record Button" class="Bool (strict)"("Val(Sgnl)"=FALSE ("Record Button")) -> ()  [unwired: 2 in, 2 out]
                }
              }
            }
            frame 1 {
              # "set cursors positions"
              n264 = Unbundle By Name(w334) -> ("Hammer cutoff"=w338:dbl, "Mic cutoff"=w337:dbl)
              n265 = call "Curtin1_SoundCardCorrection.vi"("Settings"=w334) -> ("Converted"=w332:dbl[])  [unwired: 5 in, 5 out]
              n266 = local read "View"() -> (w333:u16)
              n267 = Index Array(array=w332, index=w333) -> (element=w331:dbl)
              n268 = property on="Hammer Data" class="WFGraph (strict)"("Active Cursor"=u32 0, "Cursor.Cursor X"=w338) -> ()  [unwired: 2 in, 2 out]
              n269 = property on="Microphone Data" class="WFGraph (strict)"("Cursor.Cursor X"=w337) -> ()  [unwired: 2 in, 2 out]
              n270 = property on="Hammer Data" class="WFGraph (strict)"("Active Cursor"=u32 1, "Cursor.Cursor Y"=w331) -> ()  [unwired: 2 in, 2 out]
            }
            frame 2 {
              # "Set up plots"
              n271 = global read "Mic_Global.vi" "Last"() -> (w342:path)
              n272 = call "GetDataFiles.vi"("Settings"=w343, "View"="View", "plots"=w345, "Show history"="History", "path"=w342, "Method"="Method") -> ()  [unwired: 1 in, 5 out]
              n273 = case shown="True" "Record Button" {
                frame False {
                }
                frame True {
                  n274 = global write "Mic_Global.vi" "Task"(T5."One Shot - waiting" ("Task")) -> ()
                }
              }
            }
            frame 3 {
              # "Check for last point and redraw progress"
              n275 = property on="Progress Bar" class="Pict"() -> ("Bounds"=w348:T10)  [unwired: 2 in, 2 out]
              n276 = call "ProgressBar.vi"("Bounds"=w348, "Settings"=w347) -> ("Progress Bar"=→"Progress Bar":picture)  [unwired: 7 in, 2 out]
            }
            frame Default {
            }
          }
        }
      }
    }
  }
